vi "Global line error.vi"() -> ()   [LabVIEW 2020]
panel:
  in  "Global line error":dbl
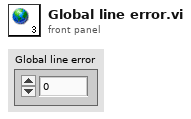
[diagram p1: front panel]
diagram:
